vi "测试-调用python处理单张图片.vi"() -> ()   [LabVIEW 2018]
panel:
  out "字符串":string
  out "Progress Bar":i32(slide) max=135 scale=1.0..2026.0
  in  "停止按钮":bool
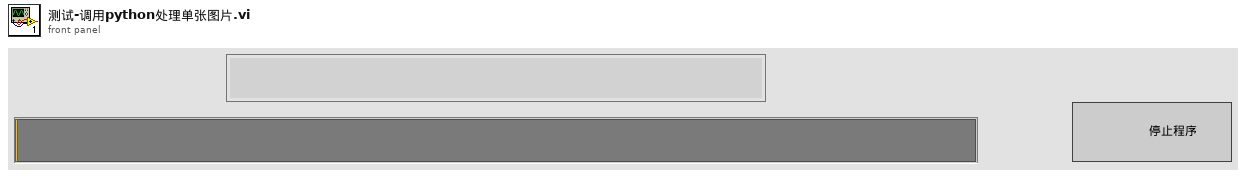
[diagram p1: front panel]
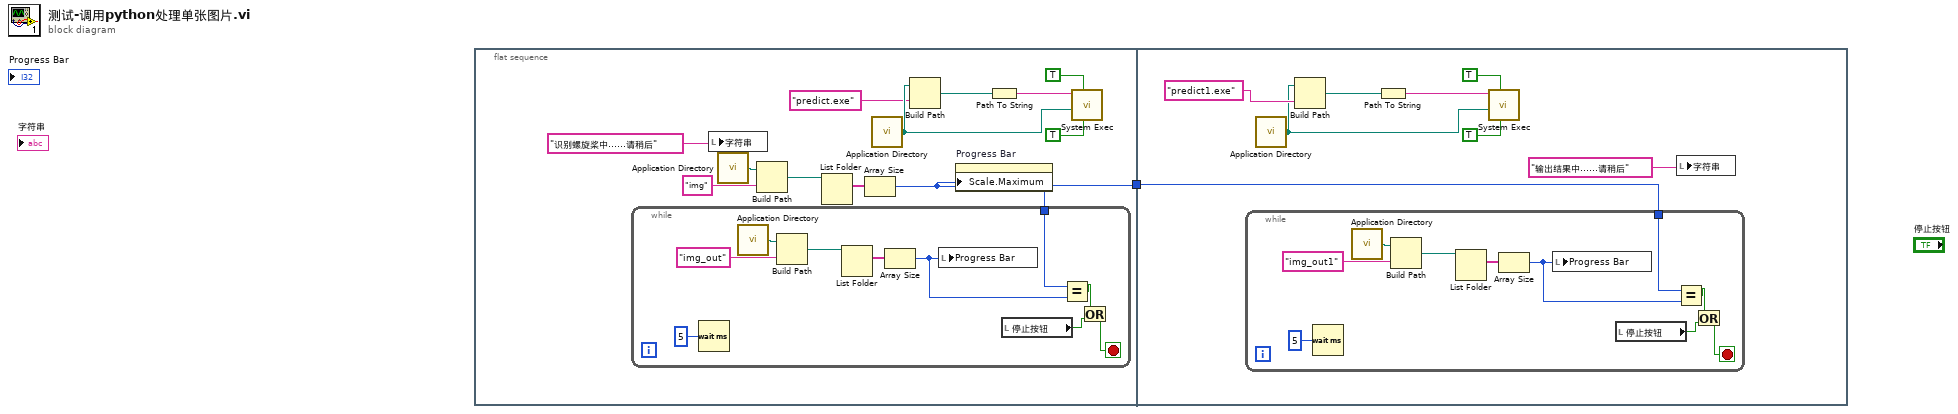
[diagram p0: block diagram]
diagram:
  n1 = flat-sequence {
    tunnel: [w2] -> w1
    tunnel: w1 -> [w24]
    frame #0 {
      n2 = local write "字符串"("识别螺旋桨中……请稍后" ("字符串")) -> ()
      n3 = call <vilib>:"Application Directory.vi"() -> ("Application Directory"=w4:path)
      n4 = Build Path(base path=w4, name or relative path="img" ("名称或相对路径")) -> (appended path=w5:path)
      n5 = List Folder(path=w5) -> (filenames=w3:string[])  [unwired: 3 in, 3 out]
      n6 = Array Size(array=w3) -> (size(s)=w2:i32)
      n7 = while {
        tunnel: w2 -> [w17]
        stop <- w14 stop-if-true
        n8 = Wait (ms)(milliseconds to wait=u32 5 ("等待时间（毫秒）")) -> ()  [unwired: 1 out]
        n9 = call <vilib>:"Application Directory.vi"() -> ("Application Directory"=w22:path)
        n10 = Build Path(base path=w22, name or relative path="img_out" ("名称或相对路径")) -> (appended path=w21:path)
        n11 = List Folder(path=w21) -> (filenames=w23:string[])  [unwired: 3 in, 3 out]
        n12 = Array Size(array=w23) -> (size(s)=w18:i32)
        n13 = local write "Progress Bar"(w18) -> ()
        n14 = local read "停止按钮"() -> (w16:bool)
        n15 = Equal?(x=w17, y=w18) -> (x = y?=w15:bool)
        n16 = Or(x=w15, y=w16) -> (x .or. y?=w14:bool)
      }
      n17 = call <vilib>:"Application Directory.vi"() -> ("Application Directory"=w11:path)
      n18 = Build Path(base path=w11, name or relative path="predict.exe" ("名称或相对路径")) -> (appended path=w9:path)
      n19 = property on="Progress Bar" class="Slide (严格)"("Scale.Maximum"=w2) -> ()  [unwired: 2 in, 2 out]
      n20 = Path To String(path=w9) -> (string=w8:string)
      n21 = call <vilib>:"System Exec.vi"("run minimized? (F)"=TRUE, "wait until completion? (T)"=TRUE, "working directory"=w11, "command line"=w8) -> ()  [unwired: 4 in, 4 out]
    }
    frame #1 {
      n22 = while {
        tunnel: w24 -> [w35]
        stop <- w32 stop-if-true
        n23 = Wait (ms)(milliseconds to wait=u32 5 ("等待时间（毫秒）")) -> ()  [unwired: 1 out]
        n24 = call <vilib>:"Application Directory.vi"() -> ("Application Directory"=w40:path)
        n25 = Build Path(base path=w40, name or relative path="img_out1" ("名称或相对路径")) -> (appended path=w39:path)
        n26 = List Folder(path=w39) -> (filenames=w41:string[])  [unwired: 3 in, 3 out]
        n27 = Array Size(array=w41) -> (size(s)=w36:i32)
        n28 = local write "Progress Bar"(w36) -> ()
        n29 = local read "停止按钮"() -> (w34:bool)
        n30 = Equal?(x=w35, y=w36) -> (x = y?=w33:bool)
        n31 = Or(x=w33, y=w34) -> (x .or. y?=w32:bool)
      }
      n32 = call <vilib>:"Application Directory.vi"() -> ("Application Directory"=w26:path)
      n33 = Build Path(base path=w26, name or relative path="predict1.exe" ("名称或相对路径")) -> (appended path=w28:path)
      n34 = Path To String(path=w28) -> (string=w27:string)
      n35 = call <vilib>:"System Exec.vi"("run minimized? (F)"=TRUE, "wait until completion? (T)"=TRUE, "working directory"=w26, "command line"=w27) -> ()  [unwired: 4 in, 4 out]
      n36 = local write "字符串"("输出结果中……请稍后" ("字符串")) -> ()
    }
  }
